vi "counter_heading.vi"() -> (0 "index":i32, 1 "counter":i32)   [LabVIEW 2009]
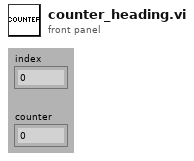
[diagram p1: front panel]
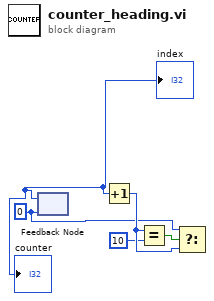
[diagram p0: block diagram]
diagram:
  w3 = 0 ("index")
  n1 = feedback #1(w3) -> (w6:i32)
  "counter" <- w6
  "index" <- w6
  n2 = Increment(x=w6) -> (x+1=w5:i32)
  n3 = Equal?(x=w5, y=10) -> (x = y?=w2:bool)
  n4 = Select(t=w3, s=w2, f=w5) -> (s? t:f=w4:i32)
